vi "CSM - Unregister Broadcast.vi"(0 "CSM Name":string, 5 "Source CSM Name (* as Default)":string="*", 7 "Status":string, 9 "Response Message (\"*\" as Default)":string="*", 11 "Error In":errorcluster caption="error in (no error)") -> (4 "CSM Name (Dup)":string, 15 "error out":errorcluster)   [LabVIEW 2017, in "Communicable State Machine.lvlib"]
doc: "### CSM - Unregister Status Change.vi\n\nUnregister notifications of status changes from other CSM modules.\n\n-- <b>Controls</b> --\n- <b>CSM Name</b>: Name of the CSM module.\n- <b>Source CSM Name</b>: The CSM module generating the status. You can use \"*\" to denote all modules generating the same status.\n- <b>Status</b>: Status string.\n\n-- <b>Indicators</b> --\n- <b>CSM Name (dup)</b>: Returns <b>CSM Name</b>."
uses:
  Communicable State Machine.lvlib
  _Support/FGV-BroadcastRegistry/Operation-BroadcastRegistry.ctl
  _Support/GlobalEvent/GEvt-Generate with Rule Check.vi
  _Support/GlobalEvent/GEvt-Convert Filter Rules - v1.0.vi
  _Support/ChangeFlag/FlagInstance-GEvt Filter.vi
  _Support/ChangeFlag/ChangeFlag-Read.vi
  _Support/GlobalEvent/LogFilter/LogFilter - Check.vi
  _Support/GlobalEvent/LogFilter/SettingVIs/Set CSM StateType Filter.vi
  _Support/GlobalEvent/LogFilter/SettingVIs/Set Global StateType Filter.vi
  _Support/GlobalEvent/LogFilter/SettingVIs/Set CSM State Filter.vi
  _Support/GlobalEvent/LogFilter/SettingVIs/Set CSM LogType Filter.vi
  _Support/GlobalEvent/LogFilter/SettingVIs/Set Global State Filter.vi
  _Support/GlobalEvent/LogFilter/SettingVIs/Set Global LogType Filter.vi
  _Support/GlobalEvent/LogFilter/SettingVIs/Set Global CSM Filter.vi
  _Support/GlobalEvent/FGV-GEvt Filter Rules(lvlibp).vi
  _Support/ChangeFlag/ChangeFlagDB.vi
  _Support/GlobalEvent/LogFilter/LogFilter.lvclass
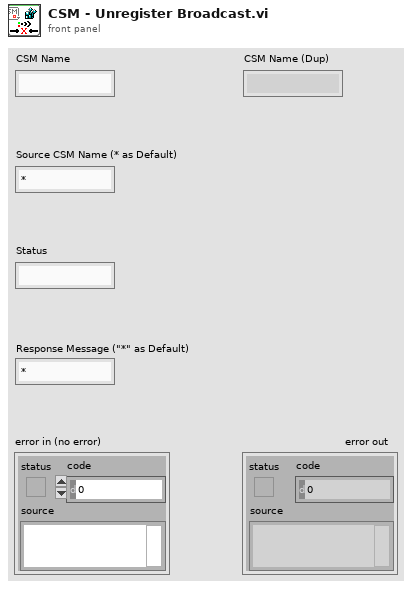
[diagram p1: front panel]
types:
  T1 = typedef "Communicable State Machine.lvlib/Operation-BroadcastRegistry.ctl" = enum16{"Delete Source Module", "Delete Target Module", "Remove Module", "Register", "Unregister", "Check", "List Status", "List Entries", "List Status Of Source", "Drop"}
  T2 = typedef "Communicable State Machine.lvlib/GEvt-Refs.ctl" = cluster{"Event":refnum<user-event>, "Queues":refnum<queue>[], "Valid":bool}
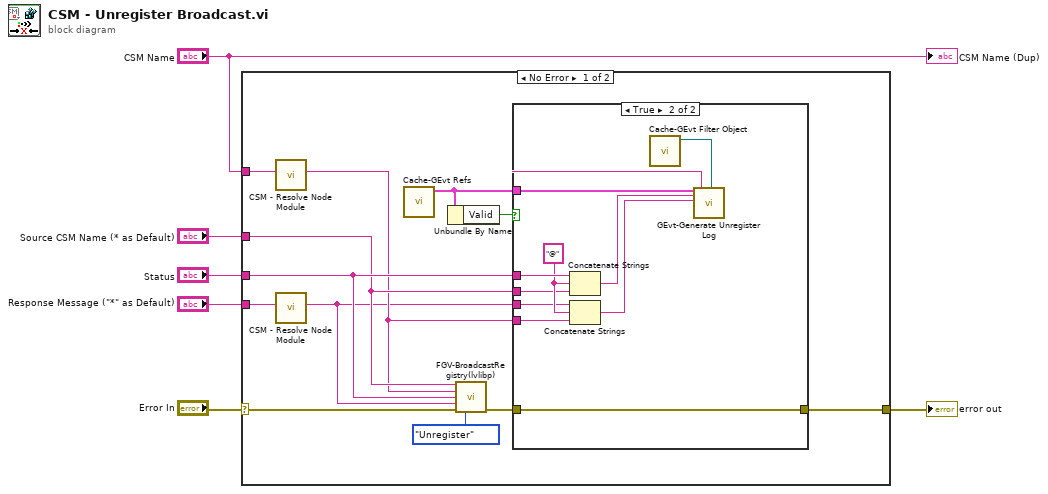
[diagram p0: block diagram]
diagram:
  n1 = case shown="No Error" "Error In" {
    selector: "Error In" -> [w17 w30]
    tunnel: [w12 w30] -> w5
    tunnel: "Response Message (\"*\" as Default)" -> [w13 _]
    tunnel: "Status" -> [w16 _]
    tunnel: "Source CSM Name (* as Default)" -> [w14 _]
    tunnel: "CSM Name" -> [w15 _]
    frame No Error {
      n2 = call "CSM - Resolve Node Module.vi"("Node Name"=w15) -> ("CSM Module Name"=w8:string)  [unwired: 10 in]
      n3 = call "CSM - Resolve Node Module.vi"("Node Name"=w13) -> ("CSM Module Name"=w7:string)  [unwired: 10 in]
      n4 = call "Cache-GEvt Refs.vi"() -> ("CSM Global Log Ref"=w10:T2)  [unwired: 10 in, 1 out]
      n5 = Unbundle By Name(w10) -> ("Valid"=w9:bool)
      n6 = call "FGV-BroadcastRegistry(lvlibp).vi"("Source"=w14, "Target"=w8, "Status"=w16, "API"=w7, "Error In"=w17, "Operation"=Operation-BroadcastRegistry."Unregister") -> ("error out"=w11:errorcluster)  [unwired: 8 in, 1 out]
      n7 = case shown="True" w9 {
        tunnel: w16 -> [_ w28]
        tunnel: w8 -> [_ w26]
        tunnel: w14 -> [_ w25]
        tunnel: w7 -> [_ w24]
        tunnel: w10 -> [_ w21]
        tunnel: [w19 w20] -> w12
        tunnel: w11 -> [w19 w20]
        frame False {
        }
        frame True {
          w27 = "@" ("string")
          n8 = Concatenate Strings(w28, w27, w25) -> (w23:string)
          n9 = Concatenate Strings(w24, w27, w26) -> (w22:string)
          n10 = call "Cache-GEvt Filter Object.vi"() -> ("CSM:LogFilter.lvclass"=w29:refnum<class "LogFilter.lvclass">)  [unwired: 11 in]
          n11 = call "GEvt-Generate Unregister Log.vi"("CSM Global Log Event"=w21, "Current State"=w23, "Arguments"=w22, "Name (\"\" to Use UUID)"=w26, "CSM:LogFilter.lvclass"=w29) -> ()  [unwired: 13 in, 2 out]
        }
      }
    }
    frame Error {
    }
  }
  "error out" <- w5
  "CSM Name (Dup)" <- "CSM Name"
